vi "oa_Extropolate Tach Pulses.vi"(7 "reset? (True)":bool, 8 "pulse buffer in":dbl[](array[numeric]), 9 "modal length":i32, 10 "extrapolation length":i32, 11 "pulse in":dbl[](array[numeric])) -> (0 "pulse buffer out":dbl[](array[numeric]), 2 "not enough pulses?":bool, 3 "pulse out":dbl[](array[numeric]))   [LabVIEW 2017, in "SoundVib_TachProcess.lvlib"]
uses:
  <vilib>/addons/Sound and Vibration/Order Analysis/Tach Process/SoundVib_TachProcess.lvlib
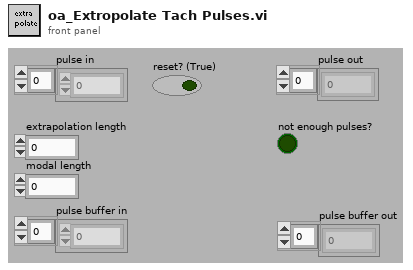
[diagram p1: front panel]
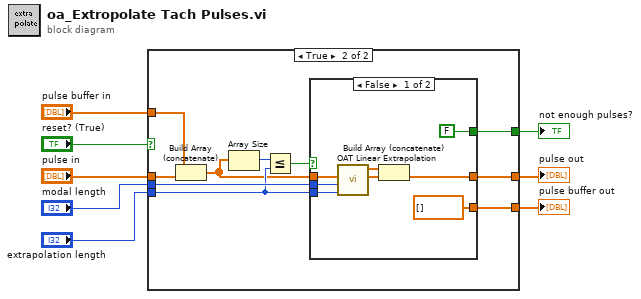
[diagram p0: block diagram]
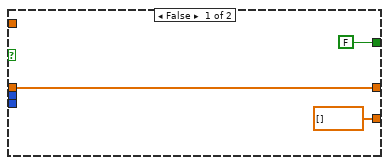
[diagram p2: hidden frame]
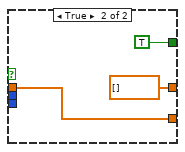
[diagram p3: hidden frame]
diagram:
  n1 = case shown="True" "reset? (True)" {
    tunnel: "pulse in" -> [w11 w15]
    tunnel: "modal length" -> [_ w21]
    tunnel: "extrapolation length" -> [_ w18]
    tunnel: [w11 w20] -> w7
    tunnel: [dbl[] [] ("Y[n]") w16] -> w8
    tunnel: "pulse buffer in" -> [_ w14]
    tunnel: [FALSE w12] -> w1
    frame False {
    }
    frame True {
      n2 = Build Array (concatenate)(w14, w15) -> (w13:dbl[])
      n3 = Array Size(array=w13) -> (size(s)=w19:i32)
      n4 = Less Or Equal?(x=w19, y=w18) -> (x <= y?=w17:bool)
      n5 = case shown="False" w17 {
        tunnel: w21 -> [w29 _]
        tunnel: [w26 dbl[] []] -> w20
        tunnel: w13 -> [w25 w31]
        tunnel: w18 -> [w24 _]
        tunnel: [dbl[] [] ("Y[n]") w31] -> w16
        tunnel: [FALSE TRUE] -> w12
        frame False {
          n6 = call <vilib>:"OAT Linear Extrapolation.vi"("extrapolation length"=w24, "modal length"=w29, "X[n]"=w25) -> ("X[n] out"=w27:dbl[], "initail"=w28:dbl[])  [unwired: 6 in, 1 out]
          n7 = Build Array (concatenate)(w28, w27) -> (w26:dbl[])
        }
        frame True {
        }
      }
    }
  }
  "pulse buffer out" <- w8
  "pulse out" <- w7
  "not enough pulses?" <- w1
